vi "Post Tweet.vi"(8 "error in (no error)":errorcluster, 10 "Tweet":string, 11 "Twitter Handle In":T1={"OAuth Credentials"={"Consumer Key"="", "Signature Method"=enum."HMAC-SHA1", "Token"="", "Version"="", "Token Secret"="", "Consumer Secret"=""}, "since ID"="", "max ID"="", "Screen Name"=""}) -> (0 "error out":errorcluster, 3 "Twitter Handle Out":T1={"OAuth Credentials"={"Consumer Key"="", "Signature Method"=enum."HMAC-SHA1", "Token"="", "Version"="", "Token Secret"="", "Consumer Secret"=""}, "since ID"="", "max ID"="", "Screen Name"=""})   [LabVIEW 2011, in "i3-twitter.lvlib"]
doc: "Post status for the authenticting user."
uses:
  i3-twitter.lvlib
  Controls/Twitter Handle.ctl
  i3-oauth/Controls/OAuth Credentials.ctl
  i3-oauth/Controls/Signature Method.ctl
  i3-oauth/Controls/HTTP Method.ctl
  <vilib>/httpClient/POSTBuffer.vi
  i3-oauth/i3-oauth.lvlib
  <vilib>/httpClient/LabVIEWHTTPClient.lvlib
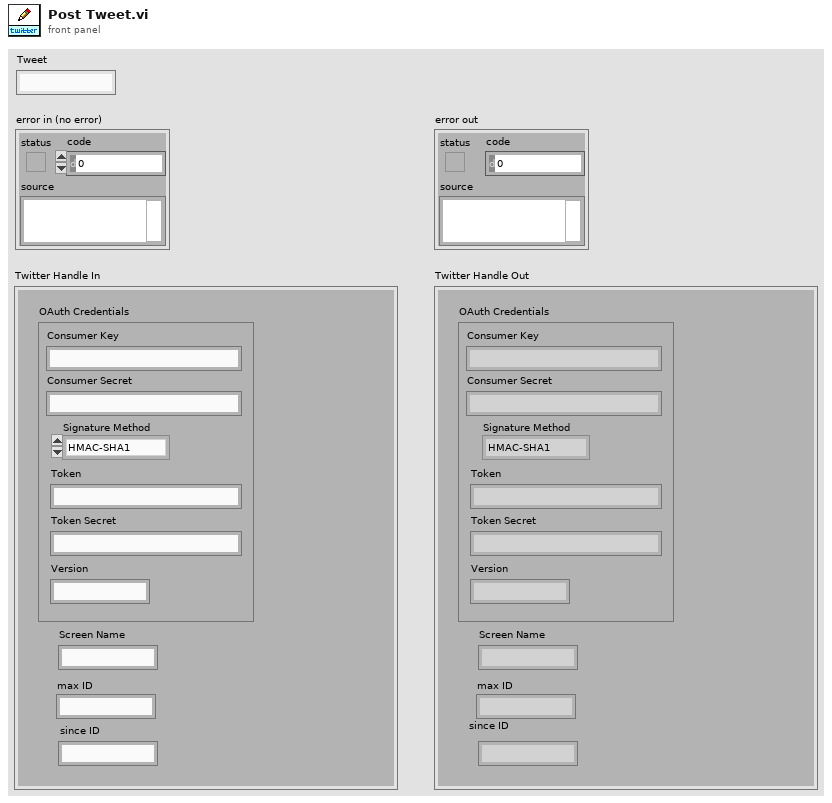
[diagram p1: front panel]
types:
  T1 = typedef "i3-twitter.lvlib/Twitter Handle.ctl" = cluster{"OAuth Credentials":T2, "since ID":string, "max ID":string, "Screen Name":string}
  T2 = typedef "i3-oauth.lvlib/OAuth Credentials.ctl" = cluster{"Consumer Key":string, "Signature Method":T3, "Token":string, "Version":string, "Token Secret":string, "Consumer Secret":string}
  T3 = typedef "i3-oauth.lvlib/Signature Method.ctl" = enum16{"HMAC-MD5", "HMAC-SHA1", "HMAC-SHA224", "HMAC-SHA256", "HMAC-SHA384", "HMAC-SHA512"}
  T4 = typedef "i3-oauth.lvlib/HTTP Method.ctl" = enum16{"GET", "POST", "PUT", "DELETE"}
  T5 = typedef "i3-oauth.lvlib/key-value-pairs.ctl" = cluster{"key":string, "value":string}
  T6 = typedef "LabVIEWHTTPClient.lvlib/ClientHandle.ctl" = refnum<k1>
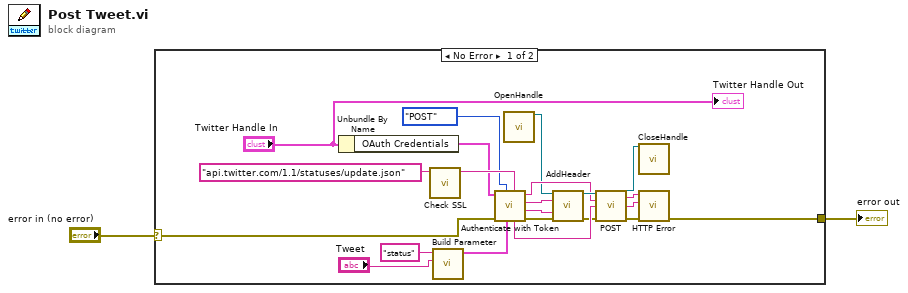
[diagram p0: block diagram]
diagram:
  n1 = case shown="No Error" "error in (no error)" {
    selector: "error in (no error)" -> [w7 w25]
    tunnel: [w12 w25] -> w2
    frame No Error {
      n2 = Unbundle By Name("Twitter Handle In") -> ("OAuth Credentials"=w3:T2)
      n3 = call "Check SSL.vi"("Input URL"="api.twitter.com/1.1/statuses/update.json" ("Base URL")) -> ("Output URL"=w5:string)  [unwired: 8 in]
      n4 = call "Build Parameter.vi"("Value"="Tweet", "Key"="status") -> ("Parameter Array"=w17:T5[])  [unwired: 9 in]
      n5 = call "Authenticate with Token.vi"("Base URL"=w5, "Body Parameters"=w17, "HTTP Method"=HTTP_Method."POST", "error in (no error)"=w7, "OAuth Credentials"=w3) -> ("error out"=w9:errorcluster, "Header Value"=w22:string, "Header Parameter"=w21:string, "Full URL"=w18:string, "Body"=w19:string)  [unwired: 2 in]
      n6 = call <vilib>:"OpenHandle.vi"() -> ("client handle out"=w11:T6)  [unwired: 14 in, 1 out]
      n7 = call <vilib>:"AddHeader.vi"("client handle"=w11, "header"=w21, "value"=w22, "error in (no error)"=w9) -> ("client handle out"=w20:T6, "error out"=w8:errorcluster)  [unwired: 10 in]
      n8 = call-poly <vilib>:"POST.vi"("client handle"=w20, "url"=w18, "data"=w19, "error in (no error)"=w8) -> ("client handle out"=w10:T6, "headers"=w15:string, "body"=w14:string, "error out"=w13:errorcluster)  [unwired: 8 in]
      n9 = call <vilib>:"CloseHandle.vi"("client handle"=w10) -> ()  [unwired: 14 in, 1 out]
      n10 = call "HTTP Error.vi"("error in (no error)"=w13, "Body"=w14, "Header"=w15) -> ("error out"=w12:errorcluster)  [unwired: 6 in, 2 out]
      "Twitter Handle Out" <- "Twitter Handle In"
    }
    frame Error {
    }
  }
  "error out" <- w2
